vi "Serial_Manager_Ophir.vi"(7 "Job":T1(ring), 8 "error in":errorcluster, 10 "write buffer":string, 11 "VISA resource":refnum<visa-resource-name>) -> (0 "error out":errorcluster, 2 "read buffer":string)   [LabVIEW 2012]
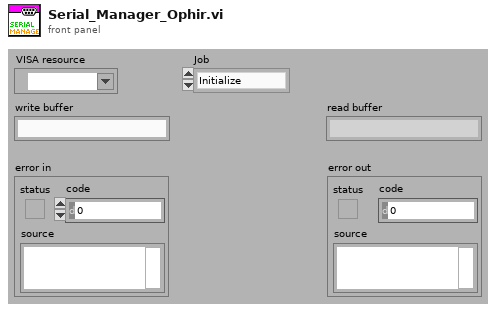
[diagram p1: front panel]
types:
  T1 = enum16{"Initialize", "Write", "Write/Read", "Read", "Clear", "Close"}
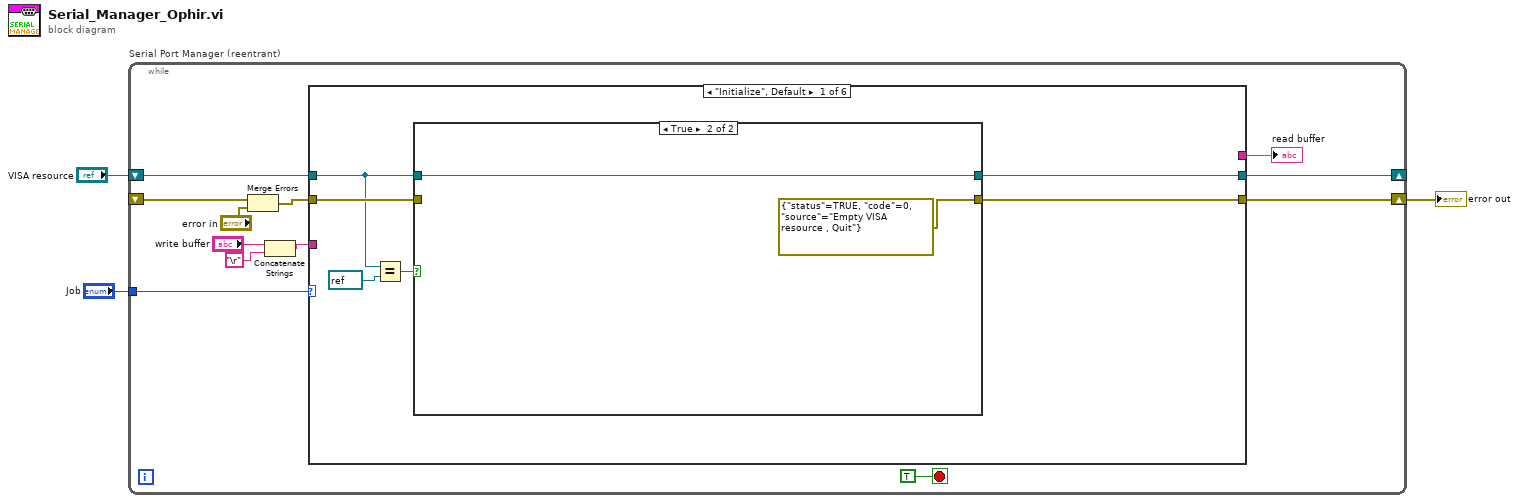
[diagram p0: block diagram]
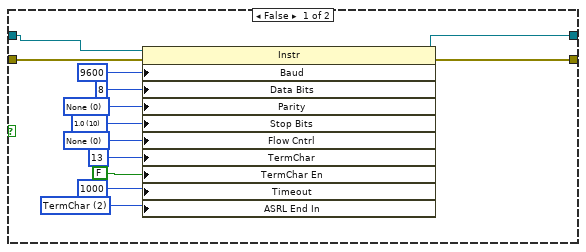
[diagram p2: hidden frame]
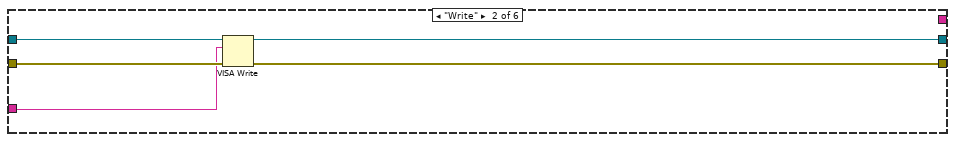
[diagram p3: hidden frame]
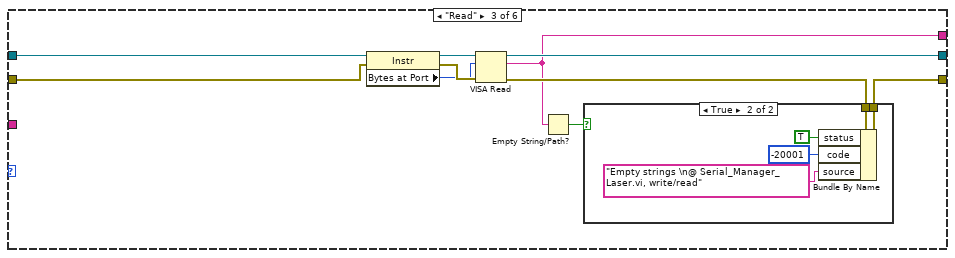
[diagram p4: hidden frame]
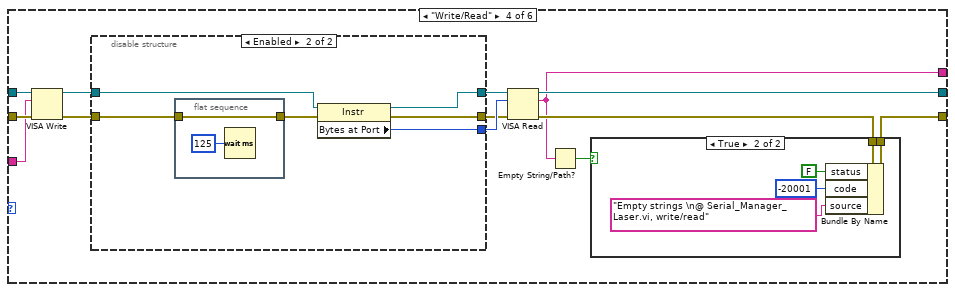
[diagram p6: hidden frame]
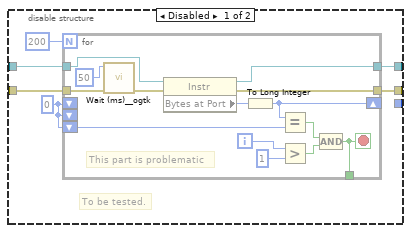
[diagram p8: hidden frame]
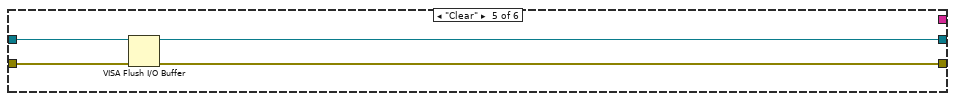
[diagram p9: hidden frame]
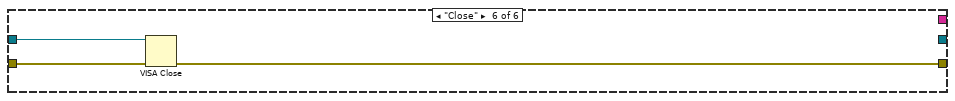
[diagram p10: hidden frame]
diagram:
  n1 = while "Serial Port Manager (reentrant)" {
    shift-right: [w14] -> _
    shift-left: "VISA resource" -> [w15]
    tunnel: "Job" -> [w13]
    shift-right: [w5] -> w1
    shift-left: _ -> [w10]
    stop <- TRUE stop-if-true
    n2 = Merge Errors(w10, "error in") -> (w11:errorcluster)
    n3 = Concatenate Strings("write buffer", "\r") -> (w7:string)
    n4 = case shown="\"Initialize\", Default" w13 {
      tunnel: w15 -> [w17 w41 w50 w68 w107 w111]
      tunnel: [w20 w38 w51 w70 w106 _] -> w14
      tunnel: [w21 w39 w44 w59 w105 w110] -> w5
      tunnel: w11 -> [w19 w40 w48 w67 w108 w109]
      tunnel: w7 -> [_ w37 _ w64 _ _]
      tunnel: [_ _ w42 w58 _ _] -> w4
      frame "Initialize", Default {
        n5 = Equal?(x=w17, y=refnum<visa-resource-name> refnum ("VISA resource")) -> (x = y?=w16:bool)
        n6 = case shown="True" w16 {
          tunnel: [w34 errorcluster {"status"=TRUE, "code"=0, "source"="Empty VISA resource , Quit"} ("error out")] -> w21
          tunnel: [w33 w36] -> w20
          tunnel: w19 -> [w25 _]
          tunnel: w17 -> [w22 w36]
          frame False {
            w24 = u16 2 items=["None", "Last Bit", "TermChar"] ("Serial Settings:End Mode for Reads")
            w28 = u16 0 items=["None", "XON/XOFF", "RTS/CTS", "XON/XOFF & RTS/CTS", "DTR/DSR", "XON/XOFF & DTR/DSR"] ("Serial Settings:Flow Control")
            w29 = u16 10 items=["1.0"=10, "1.5"=15, "2.0"=20] ("Serial Settings:Stop Bits")
            w30 = u16 0 items=["None", "Odd", "Even", "Mark", "Space"] ("Serial Settings:Parity")
            n7 = property class="Instr"(reference=w22, error in=w25, "Baud"=u32 9600 ("Serial Settings:Baud Rate"), "Data Bits"=u16 8 ("Serial Settings:Data Bits"), "Parity"=w30, "Stop Bits"=w29, "Flow Cntrl"=w28, "TermChar"=u8 13 ("Message Based Settings:Termination Character"), "TermChar En"=FALSE ("Message Based Settings:Termination Character Enable"), "Timeout"=u32 1000 ("VISA Open timeout (0)"), "ASRL End In"=w24) -> (reference out=w33:refnum<visa-resource-name>, error out=w34:errorcluster)
          }
          frame True {
          }
        }
      }
      frame "Write" {
        n8 = VISA Write(VISA resource name=w41, write buffer=w37, error in (no error)=w40) -> (VISA resource name out=w38:refnum<visa-resource-name>, error out=w39:errorcluster)  [unwired: 1 out]
      }
      frame "Read" {
        n9 = property class="Instr"(reference=w50, error in=w48) -> (reference out=w49:refnum<visa-resource-name>, error out=w47:errorcluster, "Bytes at Port"=w46:u32)
        n10 = VISA Read(VISA resource name=w49, byte count=w46, error in (no error)=w47) -> (VISA resource name out=w51:refnum<visa-resource-name>, read buffer=w42:string, error out=w43:errorcluster)  [unwired: 1 out]
        n11 = Empty String/Path?(string/path=w42) -> (empty?=w45:bool)
        n12 = case shown="True" w45 {
          tunnel: w43 -> [w52 w57]
          tunnel: [w52 w56] -> w44
          frame False {
          }
          frame True {
            n13 = Bundle By Name(cluster=w57, "status"=TRUE, "code"=-20001, "source"="Empty strings \n@ Serial_Manager_Laser.vi, write/read") -> (w56:errorcluster)
          }
        }
      }
      frame "Write/Read" {
        n14 = VISA Write(VISA resource name=w68, write buffer=w64, error in (no error)=w67) -> (VISA resource name out=w66:refnum<visa-resource-name>, error out=w65:errorcluster)  [unwired: 1 out]
        n15 = disable-structure shown="Enabled" {
          disable-tunnel: [w82 w101] -> w69
          disable-tunnel: [w81 w102] -> w62
          disable-tunnel: w66 -> [w80 w100]
          disable-tunnel: w65 -> [w79 w99]
          disable-tunnel: [_ w97] -> w63
          frame Disabled {
            w77 = 0 ("Bytes at Port")
            # "To be tested."
            n16 = for {
              N: 200 -> [_]
              tunnel: [w96] -> w82
              tunnel: [w95] -> w81
              tunnel: w80 -> [w94]
              tunnel: w79 -> [w93]
              shift-right: [w89] -> _
              shift-left: w77 -> [_]
              tunnel: [w84] -> _
              shift-left: w77 -> [_]
              shift-left: w77 -> [w83]
              i -> [w86]
              stop <- w84 stop-if-true
              # "This part is problematic"
              n17 = call <userlib>:"Wait (ms)__ogtk.vi"("error in (no error)"=w93, "milliseconds to wait"=u32 50) -> ("error out"=w92:errorcluster)  [unwired: 8 in, 1 out]
              n18 = property class="Instr"(reference=w94, error in=w92) -> (reference out=w96:refnum<visa-resource-name>, error out=w95:errorcluster, "Bytes at Port"=w90:u32)
              n19 = To Long Integer(number=w90) -> (32bit integer=w89:i32)
              n20 = Equal?(x=w89, y=w83) -> (x = y?=w88:bool)
              n21 = Greater?(x=w86, y=1) -> (0:w87:bool)
              n22 = Compound Arithmetic op=AND(w88, w87) -> (w84:bool)
            }
          }
          frame Enabled {
            n23 = flat-sequence {
              tunnel: w99 -> [w104]
              tunnel: [w104] -> w98
              frame #0 {
                n24 = Wait (ms)(milliseconds to wait=u32 125) -> ()  [unwired: 1 out]
              }
            }
            n25 = property class="Instr"(reference=w100, error in=w98) -> (reference out=w101:refnum<visa-resource-name>, error out=w102:errorcluster, "Bytes at Port"=w97:u32)
          }
        }
        n26 = VISA Read(VISA resource name=w69, byte count=w63, error in (no error)=w62) -> (VISA resource name out=w70:refnum<visa-resource-name>, read buffer=w58:string, error out=w60:errorcluster)  [unwired: 1 out]
        n27 = Empty String/Path?(string/path=w58) -> (empty?=w61:bool)
        n28 = case shown="True" w61 {
          tunnel: w60 -> [w71 w76]
          tunnel: [w71 w75] -> w59
          frame False {
          }
          frame True {
            n29 = Bundle By Name(cluster=w76, "status"=FALSE, "code"=-20001, "source"="Empty strings \n@ Serial_Manager_Laser.vi, write/read") -> (w75:errorcluster)
          }
        }
      }
      frame "Clear" {
        n30 = VISA Flush I/O Buffer(VISA resource name=w107, error in (no error)=w108) -> (VISA resource name out=w106:refnum<visa-resource-name>, error out=w105:errorcluster)  [unwired: 1 in]
      }
      frame "Close" {
        n31 = VISA Close(VISA resource name=w111, error in (no error)=w109) -> (error out=w110:errorcluster)
      }
    }
    "read buffer" <- w4
  }
  "error out" <- w1
